vi "Validate Step Action.vi"(7 "Step Number":i32, 8 "error in (no error)":errorcluster, 10 "Action in":string, 11 "Output Sequencer in":refnum<class "Output Sequencer.lvclass">) -> (0 "error out":errorcluster, 2 "Action out":string, 3 "Output Sequencer out":refnum<class "Output Sequencer.lvclass">)   [LabVIEW 2024, in "Output Sequencer.lvlib" / "Output Sequencer.lvclass"]
uses:
  Output Sequencer.lvclass
  Output Sequencer.lvclass/Output Sequencer.ctl
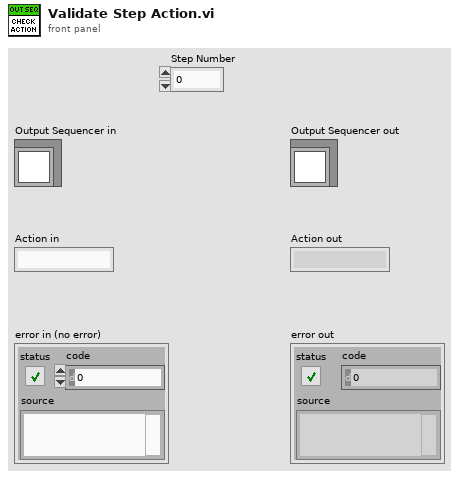
[diagram p1: front panel]
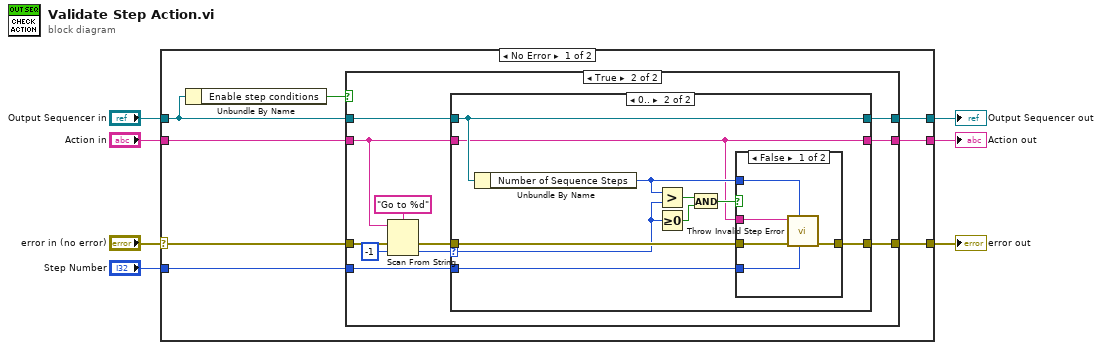
[diagram p0: block diagram]
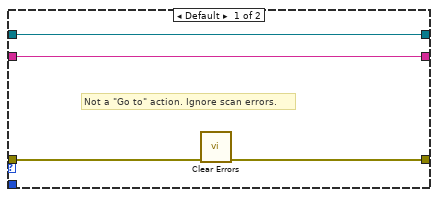
[diagram p3: hidden frame]
diagram:
  n1 = case shown="No Error" "error in (no error)" {
    selector: "error in (no error)" -> [w15 w51]
    tunnel: [w13 w51] -> w5
    tunnel: "Output Sequencer in" -> [w9 w52]
    tunnel: [w14 w52] -> w7
    tunnel: "Action in" -> [w11 w50]
    tunnel: "Step Number" -> [w12 _]
    tunnel: [w10 w50] -> w1
    frame No Error {
      n2 = Unbundle By Name(w9) -> ("Enable step conditions"=w8:bool)
      n3 = case shown="True" w8 {
        tunnel: w15 -> [w16 w27]
        tunnel: [w18 w26] -> w14
        tunnel: [w16 w23] -> w13
        tunnel: w12 -> [_ w22]
        tunnel: w11 -> [w17 w21]
        tunnel: [w17 w20] -> w10
        tunnel: w9 -> [w18 w19]
        frame False {
          # "Step conditions aren't enabled, so actions aren't used\nand we can skip validation."
        }
        frame True {
          n4 = Scan From String(format string="Go to %d", input string=w21, error in=w27, default 1=-1 ("default value 1")) -> (error out=w24:errorcluster, output 1=w25:i32)  [unwired: 1 in, 2 out]
          n5 = case shown="0.." w25 {
            selector: w25 -> [_ w37]
            tunnel: w19 -> [w33 w43]
            tunnel: [w33 w43] -> w26
            tunnel: w24 -> [w32 w41]
            tunnel: [w31 w42] -> w23
            tunnel: w21 -> [w30 w34]
            tunnel: w22 -> [_ w35]
            tunnel: [w30 w34] -> w20
            frame Default {
              # "Not a \"Go to\" action. Ignore scan errors."
              n6 = call <vilib>:"Clear Errors.vi"("error in (no error)"=w32) -> ("error out"=w31:errorcluster)  [unwired: 5 in, 1 out]
            }
            frame 0.. {
              n7 = Unbundle By Name(w43) -> ("Number of Sequence Steps"=w36:i32)
              n8 = Greater?(x=w36, y=w37) -> (0:w40:bool)
              n9 = Greater Or Equal To 0?(x=w37) -> (x >= 0?=w39:bool)
              n10 = And(x=w40, y=w39) -> (x .and. y?=w38:bool)
              n11 = case shown="False" w38 {
                tunnel: [w47 w49] -> w42
                tunnel: w41 -> [w48 w49]
                tunnel: w34 -> [w46 _]
                tunnel: w35 -> [w45 _]
                tunnel: w36 -> [w44 _]
                frame False {
                  n12 = call "Throw Invalid Step Error.vi"("Step Number"=w45, "Num Steps"=w44, "error in (no error)"=w48, "Action String in"=w46) -> ("error out"=w47:errorcluster)  [unwired: 7 in]
                }
                frame True {
                }
              }
            }
          }
        }
      }
    }
    frame Error {
    }
  }
  "Output Sequencer out" <- w7
  "error out" <- w5
  "Action out" <- w1
